vi "updateState.vi"(8 "error in (no error)":errorcluster, 10 "SWStatus":T1=enum."SettingUpState", 11 "Monochromator in":refnum<class "Monochromator.lvclass">) -> (0 "error out":errorcluster, 3 "Monochromator out":refnum<class "Monochromator.lvclass">)   [LabVIEW 2020, in "Monochromator.lvclass"]
uses:
  Monochromator.lvclass
  Typedefs/SWStatus.ctl
  MonoStateFactory/MonoStateFactory.lvclass
  Monochromator.lvclass/Monochromator.ctl
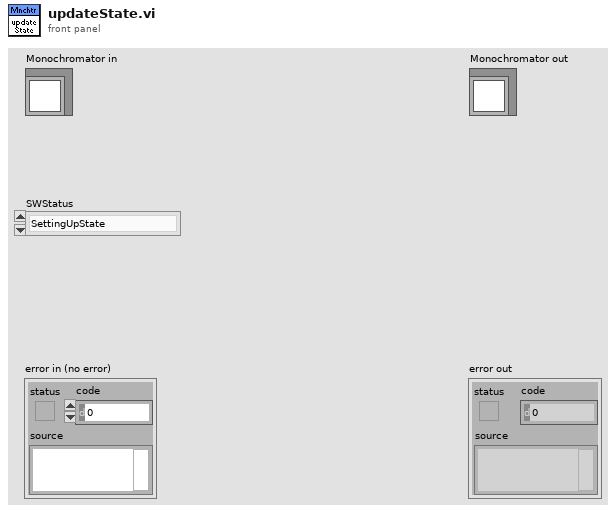
[diagram p1: front panel]
types:
  T1 = typedef "SWStatus.ctl" = enum16{"OfflineState", "ReadyState", "SettingUpState", "FaultState"}
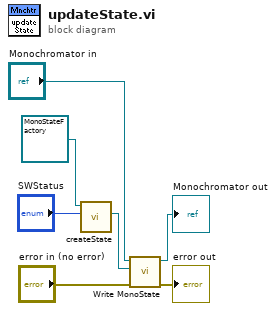
[diagram p0: block diagram]
diagram:
  n1 = call "createState.vi"("SWStatus"="SWStatus", "MonoStateFactory in"=refnum<class "MonoStateFactory.lvclass"> refnum ("MonoStateFactory.lvclass")) -> ("MonoState.lvclass"=w1:refnum<class "MonoState.lvclass">)  [unwired: 7 in, 2 out]
  n2 = call "Write MonoState.vi"("error in (no error)"="error in (no error)", "MonoState.lvclass"=w1, "Monochromator in"="Monochromator in") -> ("error out"=→"error out":errorcluster, "Monochromator out"=→"Monochromator out":refnum<class "Monochromator.lvclass">)  [unwired: 7 in]
